vi "Replication and Deployment Utility.vi"() -> ()   [LabVIEW 2013]
uses:
  subVIs/TypeDefs/rad_State Data.ctl
  subVIs/Targets/TypeDefs/rad_Targets Settings.ctl
  subVIs/Targets/TypeDefs/rad_Target Information.ctl
  subVIs/Targets/TypeDefs/rad_Target Network Settings.ctl
  subVIs/App Images/TypeDefs/rad_App Images Settings.ctl
  subVIs/App Images/TypeDefs/rad_AppImage Information.ctl
  subVIs/App Images/TypeDefs/rad_Application Image Properties.ctl
  subVIs/App Images/TypeDefs/rad_FPGA Properties.ctl
  subVIs/App Images/TypeDefs/rad_FPGA Flash Properties.ctl
  subVIs/Util/Controls/Exit Button.ctl
  subVIs/Util/Controls/Retrieve Button.ctl
  subVIs/Util/Controls/Refresh Button.ctl
  subVIs/Util/Controls/Configure Button.ctl
  subVIs/Util/Controls/Deploy Button.ctl
  subVIs/Util/Controls/Select All Button.ctl
  subVIs/Util/Controls/Add Target Button.ctl
  subVIs/Util/Controls/Compare Button.ctl
  subVIs/Util/FP Control/FP Control Functions.ctl
  <vilib>/Utility/miscctls.llb/LVRowAndColumnUnsignedTypeDef.ctl
  subVIs/RT Image Compare/TypeDefs/rad_Comparison Modes.ctl
  subVIs/rad_Globals.vi
  <vilib>/nisyscfg/Close (System).vi
  <vilib>/nisyscfg/nisyscfg.lvlib
  <resource>/objmgr/nisysapi.rc
panel:
  in  "Targets Settings":bool
  in  "Refresh Targets":T1
  in  "Target List":i32[](listbox)=[0]
  in  "Add Target":T2
  in  "Select All":T3
  in  "Configure Targets":T4
  in  "Compare":T5
  in  "Deploy":T6
  in  "Retrieve":T7
  in  "State":T8 {"Targets Information"."Primary NIC"."IP Address Request Mode" items=["Static"=1, "DHCP/Link-Local"=2, "Link-Local Only"=4, "DHCP Only"=8]}
  in  "App Images Settings":bool
  in  "Refresh Apps":T1
  in  "Exit":T17
  in  "App Images List":i32(listbox)=6
  in  "Configure App":T4
  # "Deployment Targets"
  # "Application Images"
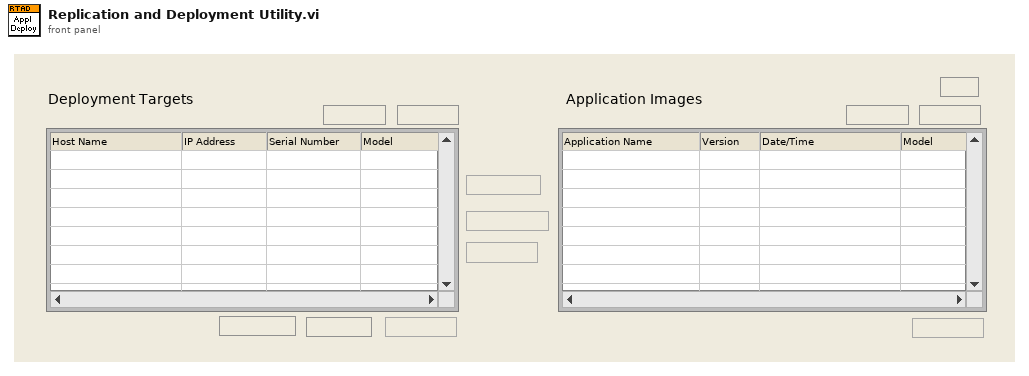
[diagram p1: front panel]
types:
  T1 = typedef "Refresh Button.ctl" = bool
  T2 = typedef "Add Target Button.ctl" = bool
  T3 = typedef "Select All Button.ctl" = bool
  T4 = typedef "Configure Button.ctl" = bool
  T5 = typedef "Compare Button.ctl" = bool
  T6 = typedef "Deploy Button.ctl" = bool
  T7 = typedef "Retrieve Button.ctl" = bool
  T8 = typedef "rad_State Data.ctl" = cluster{"Targets Settings":T9, "Targets Information":T10[], "App Images Settings":T12, "App Images Information":T13[], "Filtered Targets":i32[], "AppMode":string, "Configuration File Path":path, "Permissions":cluster{"Retrieve AppImgs":bool}, "User Added Targets":string[]}
  T9 = typedef "rad_Targets Settings.ctl" = cluster{"Target Types":string[], "Reduce Discovery Timeout":bool}
  T10 = typedef "rad_Target Information.ctl" = cluster{"Hostname":string, "Serial number":string, "Product name":string, "Product code":i32, "System status":string, "Credential type":enum16{"None/Unlocked", "FTP Password", "NIAuth Credentials"}, "User added?":bool, "Primary NIC":T11}
  T11 = typedef "rad_Target Network Settings.ctl" = cluster{"MAC address":string, "IP Address Request Mode":i32, "IP address":string, "Subnet mask":string, "Gateway":string, "DNS server":string}
  T12 = typedef "rad_App Images Settings.ctl" = cluster{"App Images Folder":path, "App Images Temp Folder":path, "CurrentVersion":string}
  T13 = typedef "rad_AppImage Information.ctl" = cluster{"AppImage Properties":T14, "AppImage Path":path}
  T14 = typedef "rad_Application Image Properties.ctl" = cluster{"Name":string, "Version":string, "Time":timestamp, "Description":string, "Key":string, "Chassis":string, "FPGA Properties":T15, "Model":string, "Retrieve":string[], "Deploy":string[], "Installed Software":string[]}
  T15 = typedef "rad_FPGA Properties.ctl" = T16[]
  T16 = typedef "rad_FPGA Flash Properties.ctl" = cluster{"Resource Name":string, "Path":path}
  T17 = typedef "Exit Button.ctl" = bool
  T18 = typedef "LVPoint32TypeDef.ctl" = cluster{"Horizontal":i32, "Vertical":i32}
  T19 = typedef "LVRowAndColumnTypeDef.ctl" = cluster{"Row":i32, "Column":i32}
  T20 = typedef "FP Control Functions.ctl" = enum16{"Open", "Close", "Bring To Front", "Center"}
  T21 = typedef "LVRowAndColumnUnsignedTypeDef.ctl" = cluster{"Row":u32, "Column":u32}
  T22 = typedef "rad_Comparison Modes.ctl" = enum32{"Compare Local Image With Controller", "Compare Two Local Images"}
  T23 = enum8{"Enabled", "Disabled", "Disabled and Grayed Out"}
  T24 = enum32{"invalid app kind", "Development System", "Run Time System", "Student Edition", "Embedded LabVIEW", "Evaluation", "Custom"}
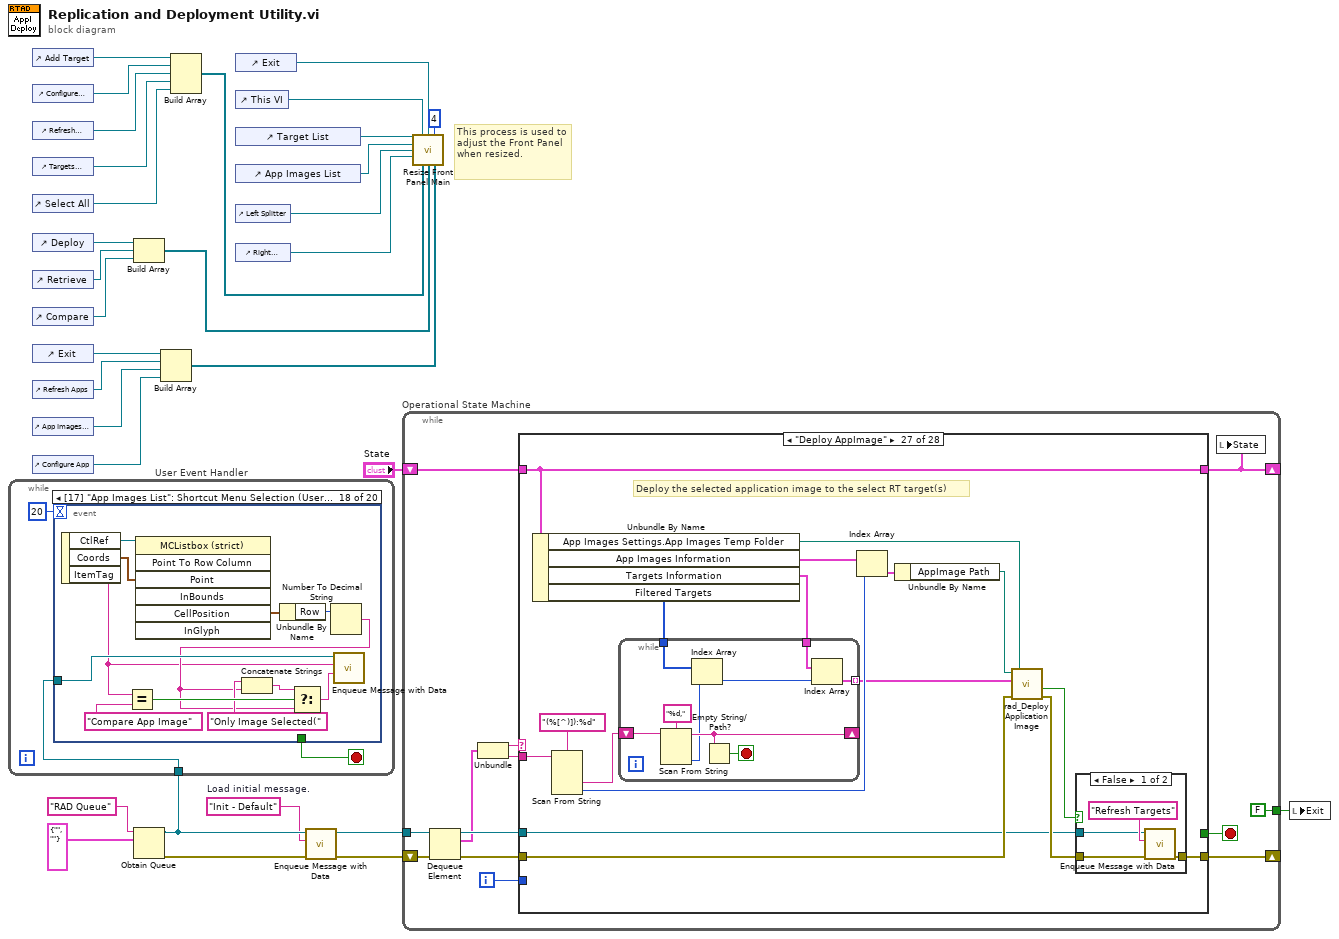
[diagram p0: block diagram]
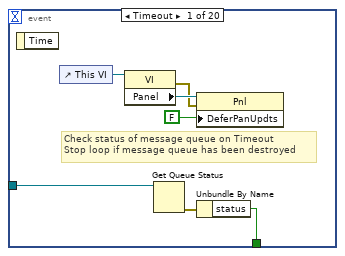
[diagram p2: hidden frame]
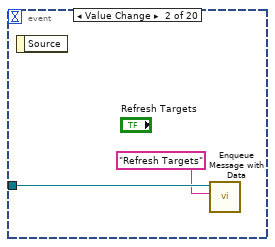
[diagram p3: hidden frame]
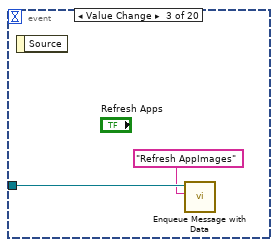
[diagram p4: hidden frame]
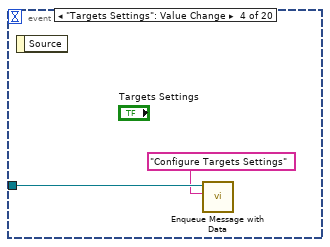
[diagram p5: hidden frame]
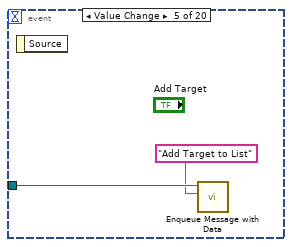
[diagram p6: hidden frame]
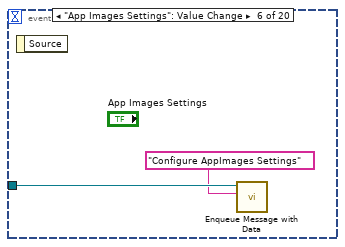
[diagram p7: hidden frame]
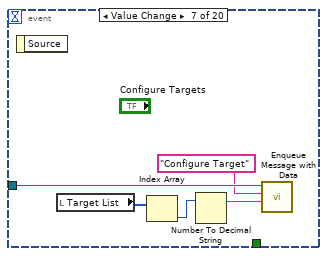
[diagram p8: hidden frame]
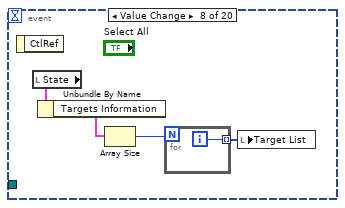
[diagram p9: hidden frame]
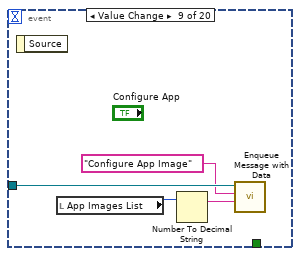
[diagram p10: hidden frame]
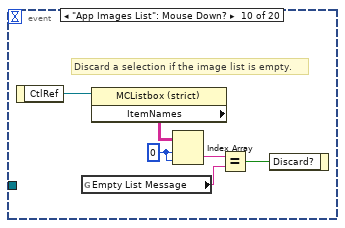
[diagram p11: hidden frame]
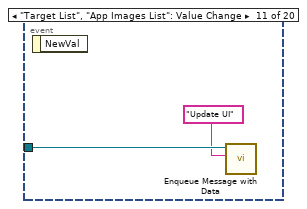
[diagram p12: hidden frame]
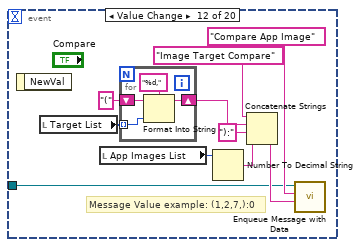
[diagram p13: hidden frame]
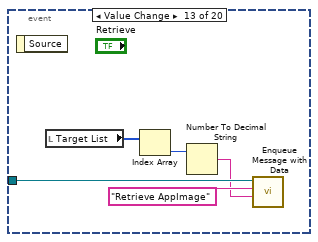
[diagram p14: hidden frame]
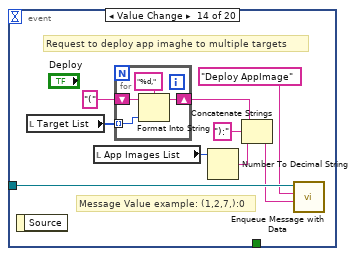
[diagram p15: hidden frame]
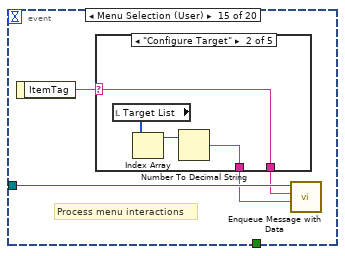
[diagram p16: hidden frame]
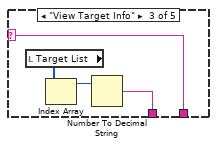
[diagram p18: hidden frame]
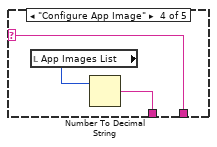
[diagram p19: hidden frame]
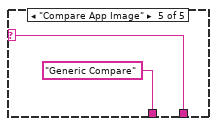
[diagram p20: hidden frame]
diagram:
  w1 = "Init - Default"  # Load initial message.
  # "This process is used to adjust the Front Panel when resized."
  n1 = control-ref of="Add Target"() -> (w22:refnum<vi>)
  n2 = control-ref of="Configure Targets"() -> (w21:refnum<vi>)
  n3 = control-ref of="Refresh Targets"() -> (w20:refnum<vi>)
  n4 = control-ref of="Targets Settings"() -> (w19:refnum<vi>)
  n5 = control-ref of="Select All"() -> (w18:refnum<vi>)
  n6 = control-ref of="Deploy"() -> (w16:refnum<vi>)
  n7 = control-ref of="Retrieve"() -> (w15:refnum<vi>)
  n8 = control-ref of="Compare"() -> (w14:refnum<vi>)
  n9 = control-ref of="Exit"() -> (w12:refnum<vi>)
  n10 = control-ref of="Refresh Apps"() -> (w11:refnum<vi>)
  n11 = control-ref of="App Images Settings"() -> (w10:refnum<vi>)
  n12 = control-ref of="Configure App"() -> (w9:refnum<vi>)
  n13 = Build Array(w16, w15, w14) -> (w13:refnum<vi>[])
  n14 = Obtain Queue(name (unnamed)="RAD Queue" ("message queue name"), element data type=cluster{string, string} {"", ""}) -> (queue out=w6:refnum<queue>, error out=w4:errorcluster)  [unwired: 3 in, 1 out]
  n15 = while "User Event Handler" {
    tunnel: w6 -> [w32]
    stop <- w33 stop-if-true
    n16 = event shown="[17] \"App Images List\": Shortcut Menu Selection (User)" {
      selector: _ -> [_ _ _ _ _ _ _ _ _ _ _ _ _ _ _ _ _ _ _ _]
      dyn-events: _ -> [_ _ _ _ _ _ _ _ _ _ _ _ _ _ _ _ _ _ _ _]
      timeout: 20 -> [_ _ _ _ _ _ _ _ _ _ _ _ _ _ _ _ _ _ _ _]
      tunnel: [w39 _ _ _ _ _ _ _ _ _ _ _ _ _ _ _ _ _ TRUE ("Discard?") w155] -> w33
      tunnel: w32 -> [w41 w43 w45 w47 w49 w51 w54 _ w64 _ w73 w76 w90 w95 w108 w126 _ w145 w151 w154]
      event Timeout {
        # "Check status of message queue on Timeout\nStop loop if message queue has been destroyed"
        n17 = event-data() -> ()  [unwired: 2 out]
        n18 = control-ref of="This VI"() -> (w35:refnum<vi>)
        n19 = property class="VI"(reference=w35) -> (error out=w36:errorcluster, "Panel"=w38:refnum<vi>)  [unwired: 1 in, 1 out]
        n20 = Get Queue Status(queue=w41) -> (error out=w40:errorcluster)  [unwired: 1 in, 8 out]
        n21 = property class="Pnl"(reference=w38, error in=w36, "DeferPanUpdts"=FALSE ("Defer Panel Updates")) -> ()  [unwired: 2 out]
        n22 = Unbundle By Name(w40) -> ("status"=w39:bool)
      }
      event Value Change {
        n23 = event-data() -> ()  [unwired: 2 out]
        n24 = call "Enqueue Message with Data.vi"("message ID"="Refresh Targets", "queue in"=w43) -> ()  [unwired: 8 in, 2 out]
      }
      event Value Change {
        n25 = event-data() -> ()  [unwired: 2 out]
        n26 = call "Enqueue Message with Data.vi"("message ID"="Refresh AppImages", "queue in"=w45) -> ()  [unwired: 8 in, 2 out]
      }
      event "Targets Settings": Value Change {
        n27 = event-data() -> ()  [unwired: 2 out]
        n28 = call "Enqueue Message with Data.vi"("message ID"="Configure Targets Settings", "queue in"=w47) -> ()  [unwired: 8 in, 2 out]
      }
      event Value Change {
        n29 = event-data() -> ()  [unwired: 2 out]
        n30 = call "Enqueue Message with Data.vi"("message ID"="Add Target to List" ("Message Name"), "queue in"=w49) -> ()  [unwired: 8 in, 2 out]
      }
      event "App Images Settings": Value Change {
        n31 = event-data() -> ()  [unwired: 2 out]
        n32 = call "Enqueue Message with Data.vi"("message ID"="Configure AppImages Settings", "queue in"=w51) -> ()  [unwired: 8 in, 2 out]
      }
      event Value Change {
        n33 = event-data() -> ()  [unwired: 2 out]
        n34 = local read "Target List"() -> (w55:i32[])
        n35 = Index Array(array=w55) -> (element=w56:i32)  [unwired: 1 in]
        n36 = Number To Decimal String(number=w56) -> (decimal integer string=w52:string)  [unwired: 1 out]
        n37 = call "Enqueue Message with Data.vi"("extra data"=w52, "message ID"="Configure Target", "queue in"=w54) -> ()  [unwired: 7 in, 2 out]
      }
      event Value Change {
        n38 = event-data() -> ()  [unwired: 2 out]
        n39 = local read "State"() -> (w59:T8)
        n40 = Unbundle By Name(w59) -> ("Targets Information"=w58:T10[])
        n41 = Array Size(array=w58) -> (size(s)=w57:i32)
        n42 = for {
          N: w57 -> [_]
          tunnel: [w61] -> w60 mode=indexing
          i -> [w61]
        }
        n43 = local write "Target List"(w60) -> ()
      }
      event Value Change {
        n44 = event-data() -> ()  [unwired: 2 out]
        n45 = local read "App Images List"() -> (w65:i32)
        n46 = Number To Decimal String(number=w65) -> (decimal integer string=w62:string)  [unwired: 1 out]
        n47 = call "Enqueue Message with Data.vi"("extra data"=w62, "message ID"="Configure App Image", "queue in"=w64) -> ()  [unwired: 7 in, 2 out]
      }
      event "App Images List": Mouse Down? {
        w69 = 0 ("index (row)")
        # "Discard a selection if the image list is empty."
        n48 = event-data() -> ("CtlRef"=w71:refnum<vi>)  [unwired: 1 out]
        n49 = global read "rad_Globals.vi" "Empty List Message"() -> (w67:string)
        n50 = property class="MCListbox (strict)"(reference=w71) -> ("ItemNames"=w70:string[][])  [unwired: 1 in, 2 out]
        n51 = Index Array(array=w70, index (row)=w69, index (col)=w69) -> (element=w68:string)
        n52 = Equal?(x=w68, y=w67) -> (x = y?=w66:bool)
        n53 = event-data("Discard?"=w66) -> ()  [unwired: 1 in, 1 out]
      }
      event "Target List", "App Images List": Value Change {
        n54 = event-data() -> ()  [unwired: 2 out]
        n55 = call "Enqueue Message with Data.vi"("message ID"="Update UI" ("Message"), "queue in"=w73) -> ()  [unwired: 8 in, 2 out]
      }
      event Value Change {
        # "Message Value example: (1,2,7,):0"
        n56 = event-data() -> ()  [unwired: 2 out]
        n57 = local read "Target List"() -> (w80:i32[])
        n58 = local read "App Images List"() -> (w79:i32)
        n59 = for {
          shift-right: [w87] -> w81
          shift-left: "(" -> [w85]
          tunnel: w80 -> [w86] mode=indexing
          n60 = Format Into String(format string="%d,", initial string=w85, w86) -> (resulting string=w87:string)  [unwired: 1 in, 1 out]
        }
        n61 = Number To Decimal String(number=w79) -> (decimal integer string=w78:string)  [unwired: 1 out]
        n62 = Concatenate Strings("Image Target Compare" ("string"), w81, "):" ("string"), w78) -> (w83:string)
        n63 = call "Enqueue Message with Data.vi"("extra data"=w83, "message ID"="Compare App Image", "queue in"=w76) -> ()  [unwired: 7 in, 2 out]
      }
      event Value Change {
        n64 = event-data() -> ()  [unwired: 2 out]
        n65 = local read "Target List"() -> (w91:i32[])
        n66 = Index Array(array=w91) -> (element=w92:i32)  [unwired: 1 in]
        n67 = Number To Decimal String(number=w92) -> (decimal integer string=w88:string)  [unwired: 1 out]
        n68 = call "Enqueue Message with Data.vi"("extra data"=w88, "message ID"="Retrieve AppImage", "queue in"=w90) -> ()  [unwired: 7 in, 2 out]
      }
      event Value Change {
        # "Request to deploy app imaghe to multiple targets"
        # "Message Value example: (1,2,7,):0"
        n69 = event-data() -> ()  [unwired: 2 out]
        n70 = local read "Target List"() -> (w97:i32[])
        n71 = local read "App Images List"() -> (w99:i32)
        n72 = for {
          shift-right: [w105] -> w96
          shift-left: "(" -> [w103]
          tunnel: w97 -> [w104] mode=indexing
          n73 = Format Into String(format string="%d,", initial string=w103, w104) -> (resulting string=w105:string)  [unwired: 1 in, 1 out]
        }
        n74 = Number To Decimal String(number=w99) -> (decimal integer string=w100:string)  [unwired: 1 out]
        n75 = Concatenate Strings(w96, "):" ("string"), w100) -> (w93:string)
        n76 = call "Enqueue Message with Data.vi"("extra data"=w93, "message ID"="Deploy AppImage", "queue in"=w95) -> ()  [unwired: 7 in, 2 out]
      }
      event Menu Selection (User) {
        # "Process menu interactions"
        n77 = event-data() -> ("ItemTag"=w109:string)  [unwired: 1 out]
        n78 = case shown="\"Configure Target\"" w109 {
          selector: w109 -> [w110 w112 w116 w120 w122]
          tunnel: [w110 w112 w116 w120 w122] -> w107
          tunnel: [_ w111 w115 w119 "Generic Compare"] -> w106
          frame Default {
          }
          frame "Configure Target" {
            n79 = local read "Target List"() -> (w114:i32[])
            n80 = Index Array(array=w114) -> (element=w113:i32)  [unwired: 1 in]
            n81 = Number To Decimal String(number=w113) -> (decimal integer string=w111:string)  [unwired: 1 out]
          }
          frame "View Target Info" {
            n82 = local read "Target List"() -> (w118:i32[])
            n83 = Index Array(array=w118) -> (element=w117:i32)  [unwired: 1 in]
            n84 = Number To Decimal String(number=w117) -> (decimal integer string=w115:string)  [unwired: 1 out]
          }
          frame "Configure App Image" {
            n85 = local read "App Images List"() -> (w121:i32)
            n86 = Number To Decimal String(number=w121) -> (decimal integer string=w119:string)  [unwired: 1 out]
          }
          frame "Compare App Image" {
          }
        }
        n87 = call "Enqueue Message with Data.vi"("extra data"=w106, "message ID"=w107, "queue in"=w108) -> ()  [unwired: 7 in, 2 out]
      }
      event "Target List": Shortcut Menu Selection (User) {
        n88 = event-data() -> ("CtlRef"=w128:refnum<vi>, "Coords"=w127:T18, "ItemTag"=w125:string)  [unwired: 2 out]
        n89 = invoke class="MCListbox (strict)" method="Point To Row Column"(reference=w128, "Point"=w127) -> ("CellPosition"=w130:T19)  [unwired: 5 in, 6 out]
        n90 = Unbundle By Name(w130) -> ("Row"=w129:i32)
        n91 = Number To Decimal String(number=w129) -> (decimal integer string=w124:string)  [unwired: 1 out]
        n92 = call "Enqueue Message with Data.vi"("extra data"=w124, "message ID"=w125, "queue in"=w126) -> ()  [unwired: 7 in, 2 out]
      }
      event "App Images List": Shortcut Menu Activation? {
        n93 = event-data() -> ("MenuRef"=w132:refnum<k9>)  [unwired: 1 out]
        n94 = global read "rad_Globals.vi" "Manager Permissions"() -> (w131:bool)
        n95 = case shown="False" w131 {
          tunnel: w132 -> [w137 _]
          tunnel: [w134 _] -> _
          frame False {
            w133 = string[] ["View App Image Info"] ("item names")
            n96 = Delete Menu Items(9:w137) -> (0:w135:errorcluster, 3:w136:refnum<k9>)  [unwired: 3 in]
            n97 = Insert Menu Items(6:w135, 7:w133, 8:w133, 9:w136) -> (0:w134:errorcluster)  [unwired: 2 in, 2 out]
          }
          frame True {
          }
        }
        n98 = event-data() -> ()  [unwired: 2 in, 1 out]
      }
      event "App Images List": Shortcut Menu Selection (User) {
        n99 = event-data() -> ("CtlRef"=w147:refnum<vi>, "Coords"=w146:T18, "ItemTag"=w138:string)  [unwired: 1 out]
        n100 = Equal?(x=w138, y="Compare App Image") -> (x = y?=w143:bool)
        n101 = invoke class="MCListbox (strict)" method="Point To Row Column"(reference=w147, "Point"=w146) -> ("CellPosition"=w149:T19)  [unwired: 5 in, 6 out]
        n102 = Unbundle By Name(w149) -> ("Row"=w148:i32)
        n103 = Number To Decimal String(number=w148) -> (decimal integer string=w140:string)  [unwired: 1 out]
        n104 = Concatenate Strings("Only Image Selected(" ("string"), w140) -> (w142:string)
        n105 = Select(t=w142, s=w143, f=w140) -> (s? t:f=w139:string)
        n106 = call "Enqueue Message with Data.vi"("extra data"=w139, "message ID"=w138, "queue in"=w145) -> ()  [unwired: 7 in, 2 out]
      }
      event Value Change {
        n107 = event-data() -> ()  [unwired: 2 out]
        n108 = call "Enqueue Message with Data.vi"("message ID"="Exit", "queue in"=w151) -> ()  [unwired: 8 in, 2 out]
      }
      event Panel Close? {
        w155 = TRUE ("Discard?")
        # "Intercepts the upper right close panel\noperation to allow a smooth shutdown\nas opposed to immediately killing the app."
        n109 = event-data() -> ()  [unwired: 2 out]
        n110 = call "Enqueue Message with Data.vi"("message ID"="Exit", "queue in"=w154) -> ()  [unwired: 8 in, 2 out]
        n111 = event-data("Discard?"=w155) -> ()  [unwired: 1 in, 1 out]
      }
    }
  }
  n112 = Build Array(w12, w11, w10, w9) -> (w8:refnum<vi>[])
  n113 = Build Array(w22, w21, w20, w19, w18) -> (w17:refnum<vi>[])
  n114 = control-ref of="Exit"() -> (w28:refnum<vi>)
  n115 = control-ref of="This VI"() -> (w27:refnum<vi>)
  n116 = control-ref of="Target List"() -> (w26:refnum<vi>)
  n117 = control-ref of="App Images List"() -> (w25:refnum<vi>)
  n118 = control-ref of="Left Splitter"() -> (w24:refnum<vi>)
  n119 = control-ref of="Right Splitter"() -> (w23:refnum<vi>)
  n120 = call "Enqueue Message with Data.vi"("error in (no error)"=w4, "message ID"=w1, "queue in"=w6) -> ("error out"=w3:errorcluster, "queue out"=w5:refnum<queue>)  [unwired: 7 in]
  n121 = while "Operational State Machine" {
    shift-left: w3 -> [w160]
    shift-right: [w161] -> _
    tunnel: w5 -> [w165]
    shift-left: "State" -> [w168]
    shift-right: [w162] -> _
    tunnel: [T17 FALSE ("Exit")] -> w7
    i -> [w164]
    stop <- w158 stop-if-true
    n122 = Dequeue Element(queue=w165, error in (no error)=w160) -> (queue out=w167:refnum<queue>, element=w163:cluster{string, string}, error out=w166:errorcluster)  [unwired: 1 in, 1 out]
    n123 = Unbundle(w163) -> (w157:string, w156:string)
    n124 = case shown="\"Deploy AppImage\"" w157 {
      tunnel: [w170 w172 w186 w214 w235 w256 w287 w302 w304 w308 w314 w326 w334 w350 w372 w388 w404 w417 w428 w430 w451 w466 w478 w486 w555 w570 w602 w618] -> w162
      tunnel: w168 -> [w170 w172 w190 w213 w236 w252 w287 w302 w304 w308 w314 w326 w335 w351 w373 w389 w404 w422 w428 w434 w452 w465 w478 w486 w555 w571 w602 w618]
      tunnel: w167 -> [_ _ w174 w196 _ w248 _ _ _ _ w321 _ w332 w346 w371 w387 _ w416 _ w432 w445 w468 _ _ w542 w574 w587 w619]
      tunnel: w166 -> [w169 w171 w179 w195 w234 w250 w284 w303 w305 w307 w320 w325 w331 w348 w367 w386 w397 w415 w427 w431 w447 w467 w479 w485 w544 w577 w590 w623]
      tunnel: w164 -> [_ _ _ _ _ _ _ _ _ _ _ _ _ _ _ _ _ _ _ _ _ _ _ _ _ _ _ _]
      tunnel: w156 -> [_ _ _ _ _ _ _ _ _ _ _ _ _ _ w381 _ w402 w426 _ _ w455 _ w475 w482 w553 w579 w601 _]
      tunnel: [w169 w171 w173 w198 w234 w249 w268 w303 w305 errorcluster {"status"=FALSE, "code"=0, "source"=""} ("error out") w315 w325 w333 w347 w369 w383 w397 w414 w427 w433 w446 w462 w479 w480 w543 w575 w589 w620] -> w161
      tunnel: [_ _ _ _ _ _ _ _ _ _ TRUE _ _ _ _ _ _ _ _ _ _ _ _ _ _ _ _ _] -> w158
      frame "Missing Message Handler", Default {
      }
      frame "**** General Application Messages ****" {
      }
      frame "Init - Default" {
        w180 = T21 {"Row"=0, "Column"=0} ("Top Left Visible Cell")
        w182 = string[][] [] ("Item Names")
        w189 = u8 2 ("Disabled")
        # "Initialize the UI"
        # "Application Folder"
        # "Default AppImages folder"
        n125 = call "Util_App Application Directory.vi"() -> ("Application Directory"=w185:path)  [unwired: 11 out]
        n126 = call "Enqueue Message with Data.vi"("error in (no error)"=w179, "message ID"="Init - Load Config", "queue in"=w174) -> ("error out"=w178:errorcluster, "queue out"=w177:refnum<queue>)  [unwired: 7 in]
        n127 = local write "App Images List"(-1 ("App Images List")) -> ()
        n128 = local write "Target List"(i32[] [] ("Target List")) -> ()
        n129 = Build Path(base path=w185, name or relative path="appimages") -> (appended path=w191:path)
        n130 = Build Path(base path=w185, name or relative path="rad_config.ini" ("Config File Name")) -> (appended path=w183:path)
        n131 = call "Enqueue Message with Data.vi"("error in (no error)"=w178, "message ID"="Init - Configure Settings", "queue in"=w177) -> ("error out"=w173:errorcluster)  [unwired: 7 in, 1 out]
        n132 = property on="Configure App" class="Bool"("Disabled"=w189) -> ()  [unwired: 2 in, 2 out]
        n133 = property on="Configure Targets" class="Bool"("Disabled"=w189) -> ()  [unwired: 2 in, 2 out]
        n134 = Bundle By Name(cluster=w190, "App Images Settings.App Images Folder"=w191, "Configuration File Path"=w183) -> (w186:T8)
        n135 = property on="Target List" class="MCListbox (strict)"("ItemNames"=w182, "TopLeft"=w180) -> ()  [unwired: 2 in, 2 out]
        n136 = property on="App Images List" class="MCListbox (strict)"("ItemNames"=w182, "TopLeft"=w180) -> ()  [unwired: 2 in, 2 out]
        n137 = call "Util_FP Control.vi"("Function"=FP_Control_Functions."Center") -> ()  [unwired: 10 in, 1 out]
      }
      frame "Init - Load Config" {
        n138 = call "rad_Load Config.vi"("error in (no error"=w195, "State in"=w213) -> ("error out"=w193:errorcluster, "State out"=w214:T8)  [unwired: 1 in, 7 out]
        n139 = call <vilib>:"Initialize Session.vi"("error in (no error)"=w193) -> ("error out"=w201:errorcluster, "Session out"=w202:refnum<k21>)  [unwired: 9 in]
        n140 = property class="System Session"(reference=w202, error in=w201) -> (reference out=w203:refnum<k21>, error out=w200:errorcluster, "InstalledVer"=w199:string)
        n141 = Scan From String(format string="%d.%d.%d", input string=w199) -> (output 1=w211:i32, output 2=w208:i32, output 3=w205:i32)  [unwired: 5 in, 3 out]
        n142 = call-poly <vilib>:"Close.vi"("error in (no error)"=w200, "Session in"=w203) -> ("error out"=w197:errorcluster)  [unwired: 9 in]
        n143 = Multiply(x=10, y=w208) -> (x*y=w206:i32)
        n144 = Multiply(x=100, y=w211) -> (x*y=w207:i32)
        n145 = Compound Arithmetic op=ADD(w207, w206, w205) -> (w204:i32)
        n146 = case shown="Default" w204 {
          tunnel: [w225 TRUE ("T button?")] -> w194
          tunnel: w197 -> [_ _]
          frame Default {
            n147 = Two Button Dialog(message="RAD requires newer functionality\nthan the software you have installed.\nPlease update to NI System Configuration\nversion 14.0 or higher.", 1:"Exit" ("F button name (\"Cancel\")"), 2:"Continue" ("T button name (\"OK\")")) -> (T button?=w225:bool)
          }
          frame 1400.. {
            # "RAD 14.0 has been fully tested\nwith NI System Configuration 14.0.\nFuture versions should work fine too."
          }
        }
        n148 = case shown="True" w194 {
          tunnel: w193 -> [w216 w223]
          tunnel: [w217 w218] -> w198
          tunnel: w196 -> [_ w222]
          frame False {
            n149 = property on="Exit" class="Bool (strict)"(error in=w216, "Val(Sgnl)"=T17 TRUE ("Value (Signaling)")) -> (error out=w217:errorcluster)  [unwired: 1 in, 1 out]
          }
          frame True {
            n150 = call "Enqueue Message with Data.vi"("error in (no error)"=w223, "message ID"="Refresh Targets", "queue in"=w222) -> ("error out"=w219:errorcluster, "queue out"=w220:refnum<queue>)  [unwired: 7 in]
            n151 = call "Enqueue Message with Data.vi"("error in (no error)"=w219, "message ID"="Refresh AppImages", "queue in"=w220) -> ("error out"=w218:errorcluster)  [unwired: 7 in, 1 out]
          }
        }
      }
      frame "Init - Configure Settings" {
        # "The temp folder should always be writable."
        # "Set permissions and update UI based on application\nmode. Disable or hide controls not appropriate\nfor current application mode."
        # "Apply configuration settings from config file"
        n152 = Unbundle By Name(w236) -> ("AppMode"=w237:string)
        n153 = case shown="\"Manager\"" w237 {
          tunnel: [TRUE ("Visible") FALSE ("Visible")] -> w233
          frame "Manager" {
          }
          frame Default {
          }
        }
        n154 = call <vilib>:"Generate Temporary File Path.vi"("Temporary File Extension (tmp)"="rad") -> ("Unique Temporary File Path"=w230:path)  [unwired: 9 in, 1 out]
        n155 = property on="Retrieve" class="Bool"("Visible"=w233) -> ()  [unwired: 2 in, 2 out]
        n156 = property on="Configure App" class="Bool"("Visible"=w233) -> ()  [unwired: 2 in, 2 out]
        n157 = Bundle By Name(cluster=w236, "App Images Settings.App Images Temp Folder"=w230, "Permissions.Retrieve AppImgs"=w233) -> (w235:T8)
        n158 = global write "rad_Globals.vi" "Manager Permissions"(w233) -> ()
        n159 = global write "rad_Globals.vi" "ShownImageVersionDialog"(FALSE ("ShownNewerVersionDialog")) -> ()
      }
      frame "Update UI" {
        # "Scroll the lists to the top if no item is selected."
        # "Display target and app images based on settings\nfor each of these tables"
        n160 = Unbundle By Name(w252) -> ("Targets Information"=w259:T10[], "Targets Settings.Target Types"=w251:string[], "App Images Information"=w253:T13[])
        n161 = call "rad_Format Application Images Information.vi"("App Images Information"=w253) -> ("App Images Information"=w254:string[][])  [unwired: 10 out]
        n162 = call "rad_FilterTargets.vi"("Target Types"=w251, "Targets Information"=w259) -> ("Filtered Targets"=w257:i32[], "Targets Information"=w258:T10[])  [unwired: 8 out]
        n163 = Bundle By Name(cluster=w252, "Filtered Targets"=w257) -> (w256:T8)
        n164 = call "rad_Format Target Information.vi"("Targets Information"=w258) -> ("Targets Information"=w255:string[][])  [unwired: 10 out]
        n165 = property on="App Images List" class="MCListbox (strict)"("ItemNames"=w254) -> (error out=w245:errorcluster)  [unwired: 2 in, 1 out]
        n166 = property on="Target List" class="MCListbox (strict)"("ItemNames"=w255) -> (error out=w246:errorcluster)  [unwired: 2 in, 1 out]
        n167 = flat-sequence {
          tunnel: w246 -> [_]
          tunnel: w245 -> [_]
          tunnel: ["App Images List"] -> w243
          tunnel: [w263] -> w244
          tunnel: [-1 ("y")] -> w241
          frame #0 {
            n168 = Array Size(array="Target List") -> (size(s)=w263:i32)
          }
        }
        n169 = Equal?(x=w243, y=w241) -> (x = y?=w240:bool)
        n170 = Equal To 0?(x=w244) -> (x = 0?=w242:bool)
        n171 = call "Enqueue Message with Data.vi"("error in (no error)"=w250, "message ID"="Update Buttons and Menus" ("Message Name"), "queue in"=w248) -> ("error out"=w249:errorcluster)  [unwired: 7 in, 1 out]
        n172 = case shown="True" w240 {
          frame False {
          }
          frame True {
            n173 = property on="App Images List" class="MCListbox (strict)"("TopLeft"=T21 {"Row"=0, "Column"=0} ("Top Left Visible Cell")) -> ()  [unwired: 2 in, 2 out]
          }
        }
        n174 = case shown="True" w242 {
          frame False {
          }
          frame True {
            n175 = property on="Target List" class="MCListbox (strict)"("TopLeft"=T21 {"Row"=0, "Column"=0} ("Top Left Visible Cell")) -> ()  [unwired: 2 in, 2 out]
          }
        }
      }
      frame "Update Buttons and Menus" {
        w272 = T23."Disabled and Grayed Out" ("Disabled")
        w273 = T23."Enabled" ("Disabled")
        # "Enable and disable buttons and \nenu items based on selections\nin both tables"
        n176 = local read "App Images List"() -> (w285:i32)
        n177 = local read "Target List"() -> (w286:i32[])
        n178 = Unbundle By Name(w287) -> ("Permissions.Retrieve AppImgs"=w266:bool)
        n179 = call "rad_Button and Menu Status.vi"("Manager Permissions"=w266, "App Image List"=w285, "Target List"=w286) -> ("Retrieve AppImage"=w276:bool, "Deploy AppImage"=w278:bool, "View Target Info"=w283:bool, "Configure App Image"=w280:bool, "Compare"=w274:bool, "Configure Target"=w282:bool)  [unwired: 3 in]
        n180 = Current VI's Menubar() -> (w288:refnum<k9>)
        n181 = Set Menu Item Info(7:"Configure Target" ("item tag"), 8:w284, 9:w282, 11:w288) -> (0:w290:errorcluster, 3:w292:refnum<k9>)  [unwired: 3 out]
        n182 = Select(t=w273, s=w282, f=w272) -> (s? t:f=w281:T23)
        n183 = Select(t=w273, s=w280, f=w272) -> (s? t:f=w279:T23)
        n184 = Select(t=w273, s=w278, f=w272) -> (s? t:f=w277:T23)
        n185 = Select(t=w273, s=w276, f=w272) -> (s? t:f=w275:T23)
        n186 = Select(t=w273, s=w274, f=w272) -> (s? t:f=w271:T23)
        n187 = Set Menu Item Info(7:"Configure App Image" ("item tag"), 8:w290, 9:w280, 11:w292) -> (0:w293:errorcluster, 3:w294:refnum<k9>)  [unwired: 3 out]
        n188 = Set Menu Item Info(7:"View Target Info" ("item tag"), 8:w293, 9:w283, 11:w294) -> (0:w295:errorcluster, 3:w296:refnum<k9>)  [unwired: 3 out]
        n189 = Set Menu Item Info(7:"Deploy AppImage" ("item tag"), 8:w295, 9:w278, 11:w296) -> (0:w297:errorcluster, 3:w298:refnum<k9>)  [unwired: 3 out]
        n190 = property on="Configure Targets" class="Bool"("Disabled"=w281) -> ()  [unwired: 2 in, 2 out]
        n191 = property on="Configure App" class="Bool"("Disabled"=w279) -> ()  [unwired: 2 in, 2 out]
        n192 = property on="Deploy" class="Bool"("Disabled"=w277) -> ()  [unwired: 2 in, 2 out]
        n193 = property on="Retrieve" class="Bool"("Disabled"=w275) -> ()  [unwired: 2 in, 2 out]
        n194 = property on="Compare" class="Bool"("DisabledEnum"=w271) -> ()  [unwired: 2 in, 2 out]
        n195 = Set Menu Item Info(7:"Retrieve AppImage" ("item tag"), 8:w297, 9:w276, 11:w298) -> (0:w269:errorcluster, 3:w270:refnum<k9>)  [unwired: 3 out]
        n196 = Set Menu Item Info(7:"Convert Images" ("item tag"), 8:w269, 9:w266, 11:w270) -> (0:w268:errorcluster)  [unwired: 4 out]
      }
      frame "Status" {
      }
      frame "About" {
        # "Show About dialog"
        n197 = call "rad_About Dialog.vi"() -> ()  [unwired: 12 out]
      }
      frame "Error" {
        # "Display run-time error message\nAdd code to log error if desired"
        n198 = disable-structure shown="TARGET_TYPE==Windows" {
          disable-tunnel: w307 -> [w309 _]
          frame condition #0 (active) {
            n199 = call <vilib>:"Simple Error Handler.vi"("error in (no error)"=w309) -> ()  [unwired: 1 in, 8 out]
          }
          frame condition #1 {
          }
        }
      }
      frame "Exit" {
        # "Store current settings in the application config file"
        # "Close the front panel if the application is running as an EXE"
        n200 = Release Queue(queue=w321, force destroy? (F)=TRUE, error in (no error)=w320) -> (error out=w313:errorcluster)  [unwired: 2 out]
        n201 = Open Application Reference() -> (0:w318:errorcluster, 3:w319:refnum<vi>)  [unwired: 4 in]
        n202 = call "rad_Save Config.vi"("error in (no error"=w313, "State"=w314) -> ("error out"=w312:errorcluster)  [unwired: 1 in, 8 out]
        n203 = property class="App"(reference=w319, error in=w318) -> ("App.Kind"=w317:T24)  [unwired: 2 out]
        n204 = case shown="\"Run Time System\"" w317 {
          frame Default {
          }
          frame "Run Time System" {
            # "Close FP in EXE"
            n205 = Current VI's Path() -> (path=w324:path)
            n206 = Open VI Reference(vi path=w324) -> (vi reference=w323:refnum<vi>, error out=w322:errorcluster)  [unwired: 5 in]
            n207 = invoke class="VI" method="FP.Close"(reference=w323, error in=w322) -> ()  [unwired: 1 in, 3 out]
          }
        }
        n208 = property on="Exit" class="Bool (strict)"(error in=w312, "Val(Sgnl)"=TRUE) -> (error out=w315:errorcluster)  [unwired: 1 in, 1 out]
      }
      frame "**** Target Messages ****" {
      }
      frame "Refresh Targets" {
        # "Refresh list of RT targets on the local subnet.\nShow progress dialog during this process."
        n209 = Unbundle By Name(w335) -> ("Targets Settings.Reduce Discovery Timeout"=w328:bool, "User Added Targets"=w341:string[], "Targets Settings.Target Types"=w327:string[])
        n210 = call "Util_Progress Show Progress Popup.vi"("error in (no error)"=w331, "Title"="Discovering Targets", "Message"="Refreshing target list...") -> ("error out"=w329:errorcluster)  [unwired: 1 in, 7 out]
        n211 = Search 1D Array(1D array=w327, element="User Targets Only") -> (index of element=w338:i32)  [unwired: 1 in]
        n212 = Not Equal?(x=w338, y=-1) -> (x != y?=w336:bool)
        n213 = call "rad_Refresh Target Information.vi"("Reduce Discovery Timeout"=w328, "error in (no error)"=w329, "User Added Targets Only"=w336, "User Added Targets"=w341) -> ("error out"=w330:errorcluster, "Targets Information"=w340:T10[])  [unwired: 6 in]
        n214 = call "Util_Progress Close Progress Popup.vi"("error in (no error)"=w330) -> ()  [unwired: 2 in, 9 out]
        n215 = Bundle By Name(cluster=w335, "Targets Information"=w340) -> (w334:T8)
        n216 = call "Enqueue Message with Data.vi"("error in (no error)"=w330, "message ID"="Update UI", "queue in"=w332) -> ("error out"=w333:errorcluster)  [unwired: 7 in, 1 out]
      }
      frame "Add Target to List" {
        n217 = Unbundle By Name(w351) -> ("User Added Targets"=w353:string[])
        n218 = call "rad_Add Target By IP Dialog.vi"() -> ("Canceled?"=w345:bool, "IP Address"=w352:string)  [unwired: 10 in]
        n219 = case shown="False" w345 {
          tunnel: w353 -> [w361 w366]
          tunnel: w352 -> [w360 _]
          tunnel: [w362 w366] -> w349
          frame False {
            n220 = Search 1D Array(1D array=w361, element=w360) -> (index of element=w365:i32)  [unwired: 1 in]
            n221 = Build Array (concatenate)(w361, w360) -> (w359:string[])
            n222 = Not Equal?(x=w365, y=-1) -> (x != y?=w363:bool)
            n223 = Select(t=w361, s=w363, f=w359) -> (s? t:f=w362:string[])
          }
          frame True {
          }
        }
        n224 = case shown="False" w345 {
          tunnel: w348 -> [w357 w358]
          tunnel: [w356 w358] -> w347
          tunnel: w346 -> [w355 _]
          frame False {
            n225 = call "Enqueue Message with Data.vi"("error in (no error)"=w357, "message ID"="Refresh Targets" ("Message Name"), "queue in"=w355) -> ("error out"=w356:errorcluster)  [unwired: 7 in, 1 out]
          }
          frame True {
          }
        }
        n226 = Bundle By Name(cluster=w351, "User Added Targets"=w349) -> (w350:T8)
      }
      frame "Configure Target" {
        # "Update network settings/configuration of the selected RT target"
        n227 = Unbundle By Name(w373) -> ("Targets Information"=w377:T10[], "Filtered Targets"=w380:i32[])
        n228 = Decimal String To Number(string=w381) -> (number=w379:i32)  [unwired: 3 out]
        n229 = Index Array(array=w380, index=w379) -> (element=w375:i32)
        n230 = Index Array(array=w377, index=w375) -> (element=w378:T10)
        n231 = call "rad_Configure Target Dialog.vi"("Error In"=w367, "Target Information in"=w378) -> ("Error Out"=w368:errorcluster, "Target Information out"=w376:T10)  [unwired: 8 out]
        n232 = Replace Array Subset(array=w377, new element=w376, index=w375) -> (w374:T10[])
        n233 = call <vilib>:"General Error Handler.vi"("error in (no error)"=w368) -> ()  [unwired: 10 in, 5 out]
        n234 = Bundle By Name(cluster=w373, "Targets Information"=w374) -> (w372:T8)
        n235 = call "Enqueue Message with Data.vi"("error in (no error)"=w367, "message ID"="Update UI", "queue in"=w371) -> ("error out"=w369:errorcluster)  [unwired: 7 in, 1 out]
      }
      frame "Configure Targets Settings" {
        # "Update the RT Target settings >> select which types of RT targets to display in the table\nCompactRIO, PXI, FieldPoint, or Other"
        n236 = Unbundle By Name(w389) -> ("Targets Settings"=w384:T9)
        n237 = call "rad_Configure Targets Settings Dialog.vi"("Targets Settings"=w384) -> ("Targets Settings"=w385:T9)  [unwired: 10 out]
        n238 = Equal?(x=w385, y=w384) -> (x = y?=w382:bool)
        n239 = Bundle By Name(cluster=w389, "Targets Settings"=w385) -> (w388:T8)
        n240 = case shown="False" w382 {
          tunnel: w387 -> [w393 _]
          tunnel: w386 -> [w392 w394]
          tunnel: [w391 w394] -> w383
          frame False {
            n241 = call "Enqueue Message with Data.vi"("error in (no error)"=w392, "message ID"="Update UI", "queue in"=w393) -> ("error out"=w391:errorcluster)  [unwired: 7 in, 1 out]
          }
          frame True {
          }
        }
      }
      frame "View Target Info" {
        # "Display additional information about the selected RT target in a popup window"
        n242 = Unbundle By Name(w404) -> ("Targets Information"=w403:T10[], "Filtered Targets"=w401:i32[])
        n243 = Decimal String To Number(string=w402) -> (number=w400:i32)  [unwired: 3 out]
        n244 = Index Array(array=w401, index=w400) -> (element=w399:i32)
        n245 = Index Array(array=w403, index=w399) -> (element=w395:T10)
        n246 = call "rad_Get Target Info (IP).vi"("error in (no error)"=w397, "Target settings in"=w395) -> ("error out"=w396:errorcluster, "Target settings out"=w398:T10)  [unwired: 8 in]
        n247 = case shown="No Error" w396 {
          selector: w396 -> [_ w406]
          tunnel: w398 -> [w405 _]
          frame No Error {
            n248 = call "rad_Target Info Dialog.vi"("Target Information"=w405) -> ()  [unwired: 11 out]
          }
          frame Error {
            n249 = call <vilib>:"General Error Handler.vi"("error in (no error)"=w406) -> ()  [unwired: 10 in, 5 out]
          }
        }
      }
      frame "Delete Target" {
        n250 = Unbundle By Name(w422) -> ("Targets Information"=w421:T10[], "Filtered Targets"=w409:i32[], "User Added Targets"=w410:string[])
        n251 = Decimal String To Number(string=w426) -> (number=w412:i32)  [unwired: 2 in, 1 out]
        n252 = Index Array(array=w409, index=w412) -> (element=w411:i32)
        n253 = Delete From Array(array=w421, length=1, index=w411) -> (deleted portion=w419:T10[], array with subset deleted=w420:T10[])
        n254 = Index Array(array=w419) -> (element=w418:T10)  [unwired: 1 in]
        n255 = Unbundle By Name(w418) -> ("Primary NIC.IP address"=w408:string)
        n256 = Search 1D Array(1D array=w410, element=w408) -> (index of element=w425:i32)  [unwired: 1 in]
        n257 = call "Enqueue Message with Data.vi"("error in (no error)"=w415, "message ID"="Update UI" ("Message Name"), "queue in"=w416) -> ("error out"=w414:errorcluster)  [unwired: 7 in, 1 out]
        n258 = Delete From Array(array=w410, length=1, index=w425) -> (array with subset deleted=w407:string[])  [unwired: 1 out]
        n259 = Bundle By Name(cluster=w422, "Targets Information"=w420, "User Added Targets"=w407) -> (w417:T8)
      }
      frame "**** Image Messages ****" {
      }
      frame "Refresh AppImages" {
        # "Update list of application images available in the configured folder"
        n260 = Unbundle By Name(w434) -> ("App Images Settings.App Images Temp Folder"=w435:path, "App Images Settings.App Images Folder"=w439:path)
        n261 = call "Util_Progress Show Progress Popup.vi"("Title"="Refreshing App Images", "Message"="Refreshing application images list...") -> ("error out"=w438:errorcluster)  [unwired: 2 in, 7 out]
        n262 = call "rad_List Application Images.vi"("App Image Temp Folder"=w435, "error in (no error)"=w438, "App Images Folder"=w439) -> ("error out"=w437:errorcluster, "Application Images Infomration"=w436:T13[])  [unwired: 1 in, 6 out]
        n263 = Bundle By Name(cluster=w434, "App Images Information"=w436) -> (w430:T8)
        n264 = call "Util_Progress Close Progress Popup.vi"("error in (no error)"=w437) -> ()  [unwired: 2 in, 9 out]
        n265 = call "Enqueue Message with Data.vi"("error in (no error)"=w431, "message ID"="Update UI" ("Message"), "queue in"=w432) -> ("error out"=w433:errorcluster)  [unwired: 7 in, 1 out]
      }
      frame "Configure App Image" {
        # "Update additional information (name, verison, description)\nstored with the selected application image"
        n266 = Unbundle By Name(w452) -> ("App Images Settings.App Images Temp Folder"=w448:path, "App Images Information"=w454:T13[])
        n267 = Decimal String To Number(string=w455) -> (number=w450:i32)  [unwired: 3 out]
        n268 = Index Array(array=w454, index=w450) -> (element=w449:T13)
        n269 = call "rad_Configure Application Image.vi"("Temp Folder"=w448, "error in (no error)"=w447, "App Images Information"=w449) -> ("error out"=w444:errorcluster, "Cancelled"=w442:bool, "App Images Information"=w443:T13)  [unwired: 6 in]
        n270 = Replace Array Subset(array=w454, new element=w443, index=w450) -> (w453:T13[])
        n271 = case shown="False" w442 {
          tunnel: [w459 w460] -> w446
          tunnel: w445 -> [w457 _]
          tunnel: w444 -> [w456 w460]
          frame False {
            n272 = call "Enqueue Message with Data.vi"("error in (no error)"=w456, "message ID"="Refresh AppImages", "queue in"=w457) -> ("error out"=w459:errorcluster)  [unwired: 7 in, 1 out]
          }
          frame True {
          }
        }
        n273 = Bundle By Name(cluster=w452, "App Images Information"=w453) -> (w451:T8)
      }
      frame "Configure AppImages Settings" {
        # "Update the selection of the folder where application images are stored"
        n274 = Unbundle By Name(w465) -> ("App Images Settings"=w464:T12)
        n275 = call "rad_Configure App Images Settings Dialog.vi"("App Images Settings"=w464) -> ("Cancelled"=w461:bool, "App Images Settings"=w463:T12)  [unwired: 1 in, 8 out]
        n276 = case shown="False" w461 {
          tunnel: w468 -> [w472 _]
          tunnel: w467 -> [w470 w473]
          tunnel: [w469 w473] -> w462
          frame False {
            n277 = call "Enqueue Message with Data.vi"("error in (no error)"=w470, "message ID"="Refresh AppImages", "queue in"=w472) -> ("error out"=w469:errorcluster)  [unwired: 7 in, 1 out]
          }
          frame True {
          }
        }
        n278 = Bundle By Name(cluster=w465, "App Images Settings"=w463) -> (w466:T8)
      }
      frame "View App Image Info" {
        n279 = Unbundle By Name(w478) -> ("App Images Information"=w477:T13[])
        n280 = Decimal String To Number(string=w475) -> (number=w474:i32)  [unwired: 2 in, 1 out]
        n281 = Index Array(array=w477, index=w474) -> (element=w476:T13)
        n282 = call "rad_View App Image Info.vi"("App Images Information"=w476) -> ()  [unwired: 11 in]
      }
      frame "Compare App Image" {
        n283 = Scan From String(format string="%[^(]", input string=w482) -> (remaining string=w481:string, output 1=w483:string)  [unwired: 2 in, 3 out]
        n284 = case shown="\"Image Target Compare\"" w483 {
          tunnel: w486 -> [w498 w527 w533]
          tunnel: w485 -> [w495 w519 w538]
          tunnel: w481 -> [w497 w529 _]
          tunnel: [w490 w517 w537] -> w480
          frame "Image Target Compare" {
            n285 = Unbundle By Name(w498) -> ("App Images Settings.App Images Folder"=w489:path, "App Images Settings.App Images Temp Folder"=w493:path, "App Images Information"=w503:T13[], "Targets Information"=w499:T10[], "Filtered Targets"=w500:i32[])
            n286 = Scan From String(format string="(%[^)]):%d", input string=w497, error in=w495) -> (error out=w491:errorcluster, output 1=w502:string, output 2=w504:i32)  [unwired: 1 in, 4 out]
            n287 = while {
              shift-right: [w512] -> _
              shift-left: w502 -> [w514]
              tunnel: w500 -> [w509]
              tunnel: w499 -> [w507]
              tunnel: [w506] -> w496 mode=indexing
              stop <- w511 stop-if-true
              n288 = Scan From String(format string="%d,", input string=w514) -> (remaining string=w512:string, output 1=w508:i32)  [unwired: 2 in, 3 out]
              n289 = Index Array(array=w509, index=w508) -> (element=w510:i32)
              n290 = Empty String/Path?(string/path=w512) -> (empty?=w511:bool)
              n291 = Index Array(array=w507, index=w510) -> (element=w506:T10)
            }
            n292 = Index Array(array=w503, index=w504) -> (element=w501:T13)
            n293 = Index Array(array=w496) -> (element=w487:T10)  [unwired: 1 in]
            n294 = Unbundle By Name(w501) -> ("AppImage Path"=w494:path)
            n295 = call "rad_RT Image Compare Dialog.vi"("App Images Repository"=w489, "Begin Automatically? (F)"=TRUE ("Show Front Panel?"), "Temp Folder"=w493, "error in (no error)"=w491, "Operation"=rad_Comparison_Modes."Compare Local Image With Controller", "Target settings"=w487, "Original Image Path"=w494) -> ("error out"=w490:errorcluster)  [unwired: 4 in]
          }
          frame "Only Image Selected" {
            n296 = Unbundle By Name(w527) -> ("App Images Settings.App Images Folder"=w516:path, "App Images Settings.App Images Temp Folder"=w522:path, "App Images Information"=w526:T13[])
            n297 = Scan From String(format string="(%d", input string=w529, error in=w519) -> (error out=w518:errorcluster, output 1=w525:i32)  [unwired: 1 in, 3 out]
            n298 = Index Array(array=w526, index=w525) -> (element=w524:T13)
            n299 = Unbundle By Name(w524) -> ("AppImage Path"=w523:path)
            n300 = call "rad_RT Image Compare Dialog.vi"("App Images Repository"=w516, "Begin Automatically? (F)"=FALSE ("Operate Headlessly?"), "Temp Folder"=w522, "error in (no error)"=w518, "Operation"=rad_Comparison_Modes."Compare Local Image With Controller", "Target settings"=T10 {"Hostname"="", "Serial number"="", "Product name"="", "Product code"=0, "System status"="", "Credential type"=enum."None/Unlocked", "User added?"=FALSE, "Primary NIC"={"MAC address"="", "IP Address Request Mode"=0, "IP address"="", "Subnet mask"="", "Gateway"="", "DNS server"=""}}, "Original Image Path"=w523) -> ("error out"=w517:errorcluster)  [unwired: 4 in]
          }
          frame "Generic Compare", Default {
            n301 = Unbundle By Name(w533) -> ("App Images Settings.App Images Folder"=w531:path, "App Images Settings.App Images Temp Folder"=w532:path)
            n302 = call "rad_RT Image Compare Dialog.vi"("App Images Repository"=w531, "Begin Automatically? (F)"=FALSE ("Operate Headlessly?"), "Temp Folder"=w532, "error in (no error)"=w538, "Operation"=rad_Comparison_Modes."Compare Local Image With Controller", "Target settings"=T10 {"Hostname"="", "Serial number"="", "Product name"="", "Product code"=0, "System status"="", "Credential type"=enum."None/Unlocked", "User added?"=FALSE, "Primary NIC"={"MAC address"="", "IP Address Request Mode"=0, "IP address"="", "Subnet mask"="", "Gateway"="", "DNS server"=""}}, "Original Image Path"=path "") -> ("error out"=w537:errorcluster)  [unwired: 4 in]
          }
        }
      }
      frame "Delete App Image" {
        n303 = Unbundle By Name(w555) -> ("App Images Information"=w554:T13[])
        n304 = Decimal String To Number(string=w553) -> (number=w552:i32)  [unwired: 2 in, 1 out]
        n305 = Index Array(array=w554, index=w552) -> (element=w551:T13)
        n306 = Unbundle By Name(w551) -> ("AppImage Path"=w546:path, "AppImage Properties.Name"=w548:string, "AppImage Properties.Version"=w539:string)
        n307 = Concatenate Strings("Are you sure you want to delete " ("string"), w548, " version " ("string"), w539, "?" ("string")) -> (w547:string)
        n308 = Two Button Dialog(message=w547, 2:"Delete" ("button name (\"OK\")")) -> (T button?=w545:bool)  [unwired: 1 in]
        n309 = case shown="True" w545 {
          tunnel: w546 -> [_ w562]
          tunnel: w544 -> [w556 w561]
          tunnel: [w556 w559] -> w543
          tunnel: w542 -> [_ w558]
          frame False {
          }
          frame True {
            n310 = Delete(path (use dialog)=w562, error in=w561) -> (error out=w560:errorcluster)  [unwired: 3 in, 2 out]
            n311 = call "Enqueue Message with Data.vi"("error in (no error)"=w560, "message ID"="Refresh AppImages" ("Message Name"), "queue in"=w558) -> ("error out"=w559:errorcluster)  [unwired: 7 in, 1 out]
          }
        }
      }
      frame "Retrieve AppImage" {
        # "Retrieve the application image\nfrom the selected RT target."
        n312 = Unbundle By Name(w571) -> ("App Images Settings.App Images Temp Folder"=w573:path, "App Images Settings.App Images Folder"=w567:path, "Targets Information"=w563:T10[], "Filtered Targets"=w564:i32[])
        n313 = Decimal String To Number(string=w579) -> (number=w578:i32)  [unwired: 3 out]
        n314 = Index Array(array=w564, index=w578) -> (element=w580:i32)
        n315 = Index Array(array=w563, index=w580) -> (element=w565:T10)
        n316 = call "rad_Retrieve Application Image From Target.vi"("App Images Temp Folder"=w573, "error in (no error)"=w577, "Target settings"=w565, "App Images Folder"=w567) -> ("error out"=w576:errorcluster, "Cancelled"=w568:bool, "New App Image Path"=w572:path)  [unwired: 3 in, 2 out]
        n317 = Strip Path(path=w572) -> (stripped path=w569:path)  [unwired: 1 out]
        n318 = case shown="False" w568 {
          tunnel: w576 -> [w584 w585]
          tunnel: [w583 w585] -> w575
          tunnel: w574 -> [w582 _]
          frame False {
            n319 = call "Enqueue Message with Data.vi"("error in (no error)"=w584, "message ID"="Refresh AppImages" ("Message Name"), "queue in"=w582) -> ("error out"=w583:errorcluster)  [unwired: 7 in, 1 out]
          }
          frame True {
          }
        }
        n320 = Select(t=w567, s=w568, f=w569) -> (s? t:f=w566:path)
        n321 = Bundle By Name(cluster=w571, "App Images Settings.App Images Folder"=w566) -> (w570:T8)
      }
      frame "Deploy AppImage" {
        # "Deploy the selected application image to the select RT target(s)"
        n322 = Unbundle By Name(w602) -> ("App Images Settings.App Images Temp Folder"=w592:path, "App Images Information"=w598:T13[], "Targets Information"=w594:T10[], "Filtered Targets"=w595:i32[])
        n323 = Scan From String(format string="(%[^)]):%d", input string=w601) -> (output 1=w597:string, output 2=w599:i32)  [unwired: 2 in, 5 out]
        n324 = while {
          shift-right: [w614] -> _
          shift-left: w597 -> [w616]
          tunnel: w595 -> [w611]
          tunnel: w594 -> [w609]
          tunnel: [w608] -> w591 mode=indexing
          stop <- w613 stop-if-true
          n325 = Scan From String(format string="%d,", input string=w616) -> (remaining string=w614:string, output 1=w610:i32)  [unwired: 2 in, 3 out]
          n326 = Index Array(array=w611, index=w610) -> (element=w612:i32)
          n327 = Empty String/Path?(string/path=w614) -> (empty?=w613:bool)
          n328 = Index Array(array=w609, index=w612) -> (element=w608:T10)
        }
        n329 = Index Array(array=w598, index=w599) -> (element=w596:T13)
        n330 = Unbundle By Name(w596) -> ("AppImage Path"=w593:path)
        n331 = call "rad_Deploy Application Image.vi"("App Image Temp Folder"=w592, "error in (no error)"=w590, "Selected Targets"=w591, "App Image Path"=w593) -> ("error out"=w588:errorcluster, "Cancelled"=w586:bool)  [unwired: 6 out]
        n332 = case shown="False" w586 {
          tunnel: [w606 w607] -> w589
          tunnel: w588 -> [w605 w607]
          tunnel: w587 -> [w603 _]
          frame False {
            n333 = call "Enqueue Message with Data.vi"("error in (no error)"=w605, "message ID"="Refresh Targets" ("Message Name"), "queue in"=w603) -> ("error out"=w606:errorcluster)  [unwired: 7 in, 1 out]
          }
          frame True {
          }
        }
      }
      frame "Convert Images" {
        n334 = Unbundle By Name(w618) -> ("App Images Settings.App Images Folder"=w617:path)
        n335 = call "Util_ConvertImageToLatest.vi"("error in (no error)"=w623, "Image Path"=w617) -> ("error out"=w621:errorcluster)  [unwired: 9 in]
        n336 = call "Enqueue Message with Data.vi"("error in (no error)"=w621, "message ID"="Refresh AppImages" ("Message Name"), "queue in"=w619) -> ("error out"=w620:errorcluster)  [unwired: 7 in, 1 out]
      }
    }
    n337 = local write "State"(w162) -> ()
  }
  n338 = call "Resize Front Panel Main.vi"("Left Listbox"=w26, "Top Level VI"=w27, "Stop"=w28, "Number of Columns"=4, "Right Listbox"=w25, "Left Splitter"=w24, "Right Splitter"=w23, "Left Pane Items"=w17, "Mid Pane Items"=w13, "Right Pane Items"=w8) -> ()  [unwired: 5 in, 1 out]
  n339 = local write "Exit"(w7) -> ()
